vi "disdrometer_BuildWarningString.vi"(10 "UserCfg":T1, 11 "WriteChannel":string) -> (2 "WarningString":string)   [LabVIEW 2018]
uses:
  UserConfig_ChannelSettings_Clust.ctl
  NASA/te_2015/TE_ControlType_Enum.ctl
  NASA/te_2015/TE_Polarity_Enum.ctl
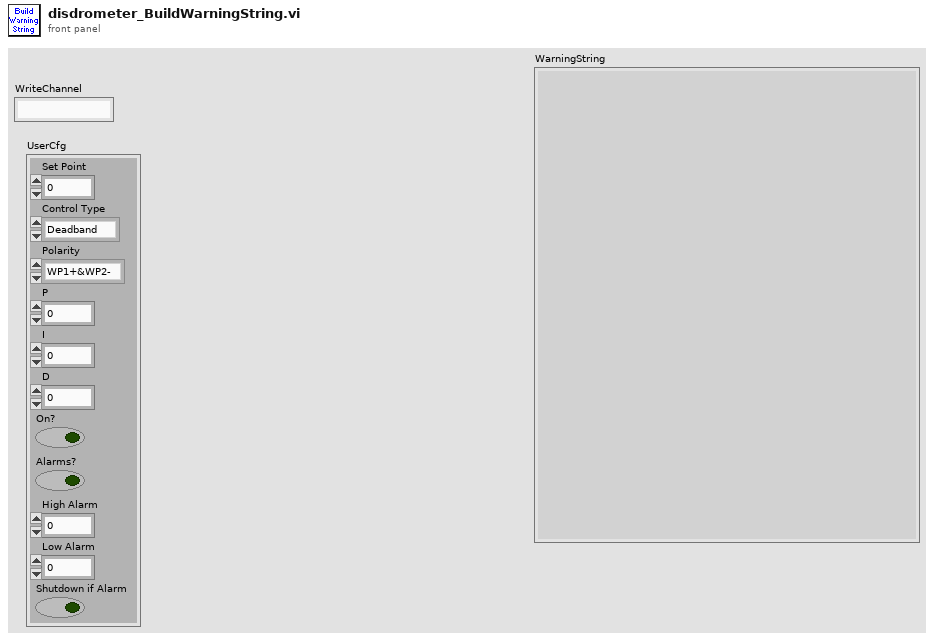
[diagram p1: front panel]
types:
  T1 = typedef "UserConfig_ChannelSettings_Clust.ctl" = cluster{"Set Point":dbl, "Control Type":T2, "Polarity":T3, "P":dbl, "I":dbl, "D":dbl, "On?":bool, "Alarms?":bool, "High Alarm":dbl, "Low Alarm":dbl, "Shutdown if Alarm":bool}
  T2 = typedef "TE_ControlType_Enum.ctl" = enum16{"Deadband", "PID", "Computer"}
  T3 = typedef "TE_Polarity_Enum.ctl" = enum16{"WP1+&WP2-", "WP2+&WP1-"}
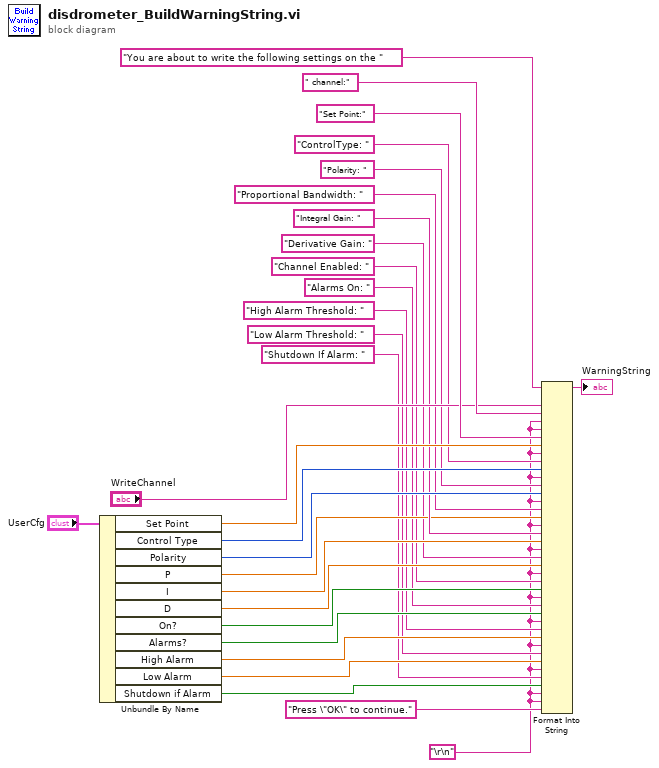
[diagram p0: block diagram]
diagram:
  w1 = "\r\n"
  n1 = Unbundle By Name("UserCfg") -> ("Set Point"=w24:dbl, "Control Type"=w22:T2, "Polarity"=w20:T3, "P"=w16:dbl, "I"=w17:dbl, "D"=w14:dbl, "On?"=w12:bool, "Alarms?"=w10:bool, "High Alarm"=w8:dbl, "Low Alarm"=w6:dbl, "Shutdown if Alarm"=w4:bool)
  n2 = Format Into String(initial string="You are about to write the following settings on the ", "WriteChannel", " channel:" ("initial string"), w1, w1, "Set Point:" ("input 4"), w24, w1, "ControlType: " ("input 4"), w22, w1, "Polarity: " ("input 4"), w20, w1, "Proportional Bandwidth: " ("input 4"), w16, w1, "Integral Gain: " ("input 4"), w17, w1, "Derivative Gain: " ("input 4"), w14, w1, "Channel Enabled: " ("input 4"), w12, w1, "Alarms On: " ("input 4"), w10, w1, "High Alarm Threshold: " ("input 4"), w8, w1, "Low Alarm Threshold: " ("input 4"), w6, w1, "Shutdown If Alarm: " ("input 4"), w4, w1, w1, "Press \"OK\" to continue." ("input 37")) -> (resulting string=→"WarningString":string)  [unwired: 2 in, 1 out]
